vi "Read Write_.vi"(8 "error in (no error)":errorcluster, 11 "Set Wvfm Write CMD in":refnum<class "Set Wvfm Write CMD.lvclass">) -> (0 "error out":errorcluster, 2 "Write?":bool, 3 "Set Wvfm Write CMD out":refnum<class "Set Wvfm Write CMD.lvclass">)   [LabVIEW 2014, in "ePAS Library.lvlib" / "Set Wvfm Write CMD.lvclass"]
uses:
  Set Wvfm Write CMD.lvclass
  Set Wvfm Write CMD.lvclass/Set Wvfm Write CMD.ctl
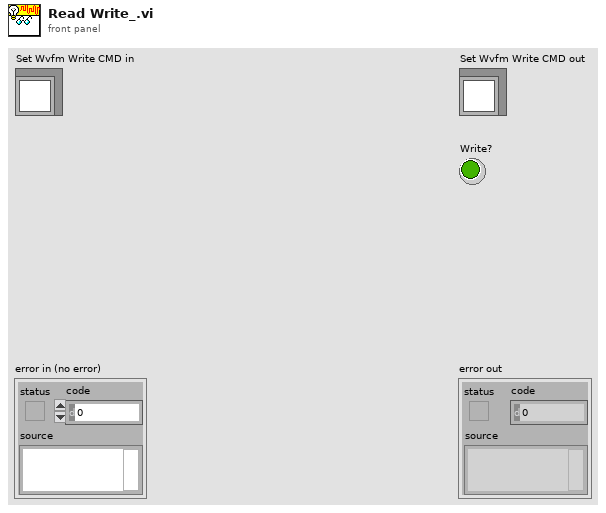
[diagram p1: front panel]
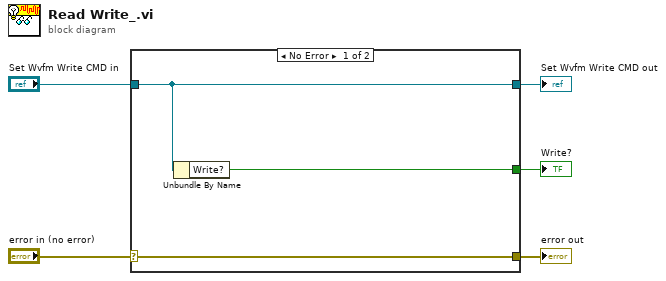
[diagram p0: block diagram]
diagram:
  n1 = case shown="No Error" "error in (no error)" {
    selector: "error in (no error)" -> [w8 w9]
    tunnel: [w8 w9] -> w4
    tunnel: [w7 w10] -> w2
    tunnel: "Set Wvfm Write CMD in" -> [w7 w10]
    tunnel: [w6 _] -> w1
    frame No Error {
      n2 = Unbundle By Name(w7) -> ("Write?"=w6:bool)
    }
    frame Error {
    }
  }
  "error out" <- w4
  "Set Wvfm Write CMD out" <- w2
  "Write?" <- w1
